vi "Actor Event Wrapper.vi"(8 "Queue Mailbox":refnum<data-value>, 9 "Self Alias":string, 10 "Queue of Event Self":refnum<queue>, 11 "Event jettl":refnum<class "Event.lvclass">) -> ()   [LabVIEW 2021, in "jettl.lvlib" / "Base Event jettl.lvlib"]
uses:
  Base Event jettl.lvlib
  Event/Event.lvclass
  Msg Strategy/Msg Strategy.lvclass
  Queue Mailbox/Queue Mailbox/Queue Mailbox.lvclass
  Base Event jettl/Base Event jettl.lvclass
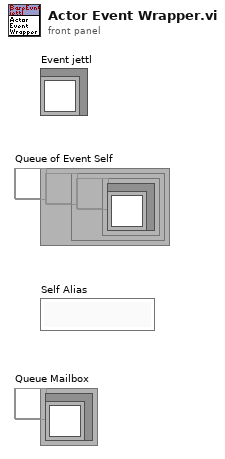
[diagram p1: front panel]
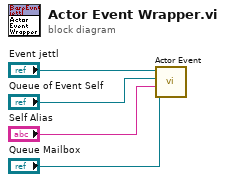
[diagram p0: block diagram]
diagram:
  n1 = call "Actor Event.vi"("Queue Mailbox"="Queue Mailbox", "Self Alias"="Self Alias", "Queue of Event Self"="Queue of Event Self", "Event jettl"="Event jettl") -> ()  [unwired: 8 in]
